vi "initRandStimAll.vi"(8 "error in (no error)":errorcluster, 11 "Stimulus in":refnum<class "Stimulus.lvclass">) -> (0 "error out":errorcluster, 3 "Stimulus out":refnum<class "Stimulus.lvclass">)   [LabVIEW 2014, in "Stimulus.lvclass"]
uses:
  Stimulus.lvclass
  Stimulus.lvclass/Stimulus.ctl
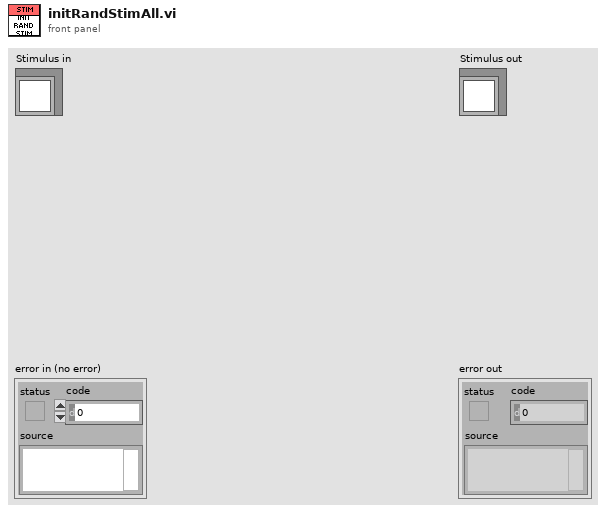
[diagram p1: front panel]
types:
  T1 = typedef "IMAQ Image.ctl" = refnum<image>
  T2 = cluster{"Image":T1, "Window Number (0...15)":i32, "Coordinates (screen)":cluster{"X Position":i32, "Y Position":i32}, "Window name":string, "Time":dbl, "Response \nperiod":dbl, "TI delay":dbl, "Punishment Delay":dbl, "Stim queue":refnum<queue>, "ExpType":enum16{"Orientation", "Calibrate", "Freerun", "BW"}, "Stimuli":string, "Rewarded Stimuli":string, "RI":dbl, "Correct response":bool, "Next Image 2":T1}[]
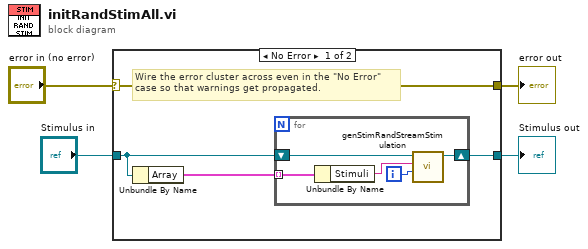
[diagram p0: block diagram]
diagram:
  n1 = case shown="No Error" "error in (no error)" {
    selector: "error in (no error)" -> [w8 w15]
    tunnel: [w8 w15] -> w3
    tunnel: [w5 w14] -> w1
    tunnel: "Stimulus in" -> [w6 w14]
    frame No Error {
      # "Wire the error cluster across even in the \"No Error\"\ncase so that warnings get propagated."
      n2 = Unbundle By Name(w6) -> ("Array"=w7:T2)
      n3 = for {
        tunnel: w7 -> [w12] mode=indexing
        shift-right: [w9] -> w5
        shift-left: w6 -> [w10]
        i -> [w13]
        n4 = Unbundle By Name(w12) -> ("Stimuli"=w11:string)
        n5 = call-dynamic "genStimRandStreamStimulation.vi"("index"=w13, "Stimuli"=w11, "Stimulus in"=w10) -> ("Stimulus out"=w9:refnum<class "Stimulus.lvclass">)  [unwired: 7 in, 1 out]
      }
    }
    frame Error {
    }
  }
  "error out" <- w3
  "Stimulus out" <- w1
